vi "CloseDevices.vi"(1 "Devices":T1[](array[typedef])) -> (0 "Devices":T1[](array[typedef]))   [LabVIEW 2010]
uses:
  Controls/SpiDevice.ctl
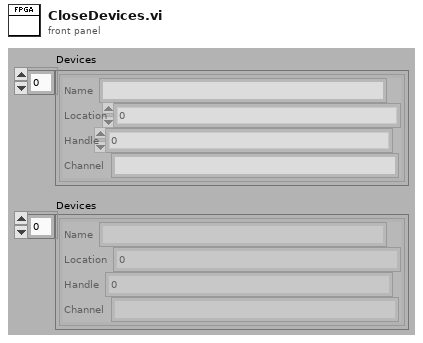
[diagram p1: front panel]
types:
  T1 = typedef "SpiDevice.ctl" = cluster{"Name":string, "Location":u32, "Handle":u32, "Channel":string}
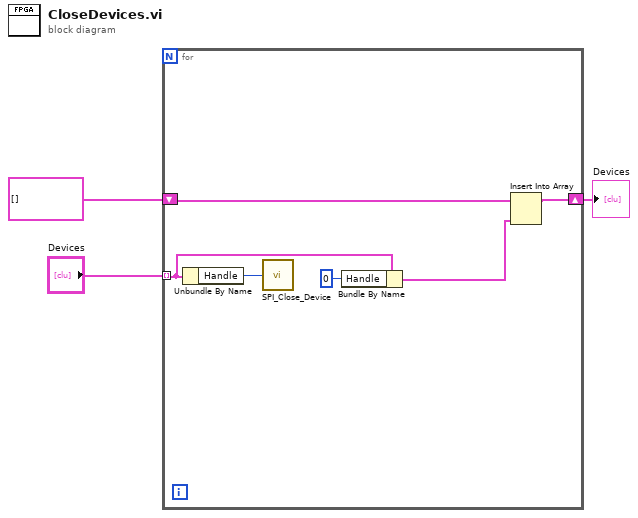
[diagram p0: block diagram]
diagram:
  n1 = for {
    tunnel: "Devices" -> [w8] mode=indexing
    shift-right: [w6] -> w1
    shift-left: T1[] [] ("Devices 2") -> [w5]
    n2 = Unbundle By Name(w8) -> ("Handle"=w9:u32)
    n3 = call "SPI_Close_Device.vi"("Handle"=w9) -> ()  [unwired: 1 out]
    n4 = Bundle By Name(cluster=w8, "Handle"=u32 0) -> (w4:T1)
    n5 = Insert Into Array(array=w5, new element=w4) -> (w6:T1[])  [unwired: 1 in]
  }
  "Devices" <- w1
